vi "Message Handling Loop - Screenpop.vi"(8 "error in":errorcluster, 9 "Message Queues in":T1, 10 "User Event Bundle":T2) -> (0 "error out":errorcluster)   [LabVIEW 2018]
uses:
  Type Defs/User Events.ctl
  Support/Message Queue/All Message Queues.ctl
  Support/Message Queue/Message Cluster.ctl
  Type Defs/Screenpop Loop Data.ctl
  Type Defs/FGV States.ctl
  <vilib>/Utility/error.llb/Error Cluster From Error Code.vi
  <vilib>/ErrorRing/Error Ring.xnode
  Support/Message Queue/Message Queue.lvlib
  Support/User Events/User Events.lvlib
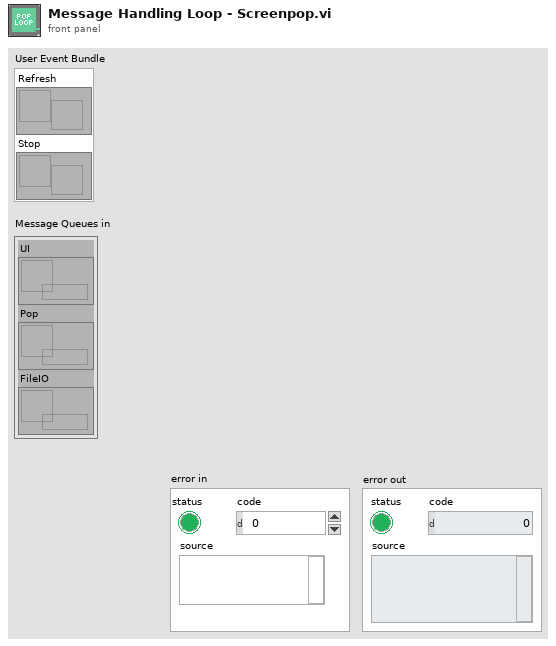
[diagram p1: front panel]
types:
  T1 = typedef "Message Queue.lvlib/All Message Queues.ctl" = cluster{"UI":refnum<queue>, "Pop":refnum<queue>, "FileIO":refnum<queue>}
  T2 = typedef "User Events.ctl" = cluster{"Refresh":refnum<user-event>, "Stop":refnum<user-event>}
  T3 = typedef "Screenpop Loop Data.ctl" = cluster{"Update List":i32[], "UI":refnum<queue>}
  T4 = typedef "FGV States.ctl" = enum16{"Initialize", "Merge", "Write", "Remove", "Read", "Clear"}
  T5 = typedef "SR Cluster.ctl" = cluster{"Color":u32, "SR Number":i32, "SR Status":T6, "Name":string, "Summary":string, "Last Updated":timestamp, "SR Type":string, "Service Level":string, "Days Open":dbl, "Creation Date":timestamp, "Owner":string, "Note":string}
  T6 = typedef "SR Status.ctl" = enum16{"Caller Abandoned", "Created in Error", "Expired", "Forum Resolved AE", "Forum Resolved Customer", "IN WORK", "IN WORK Collab with AES", "IN WORK Collab with PSE", "IN WORK Collab with SE", "IN WORK Customer Added Note", "IN WORK Escalation", "IN WORK Wait on Customer", "Open", "Potentially Resolved", "Presumed Resolved", "RMA Approved for Return", "RMA Closed", "RMA Closed - DOA", "RMA In Progress", "RMA Open", "RMA Waiting on Customer", "Resolved", "Passed Off"}
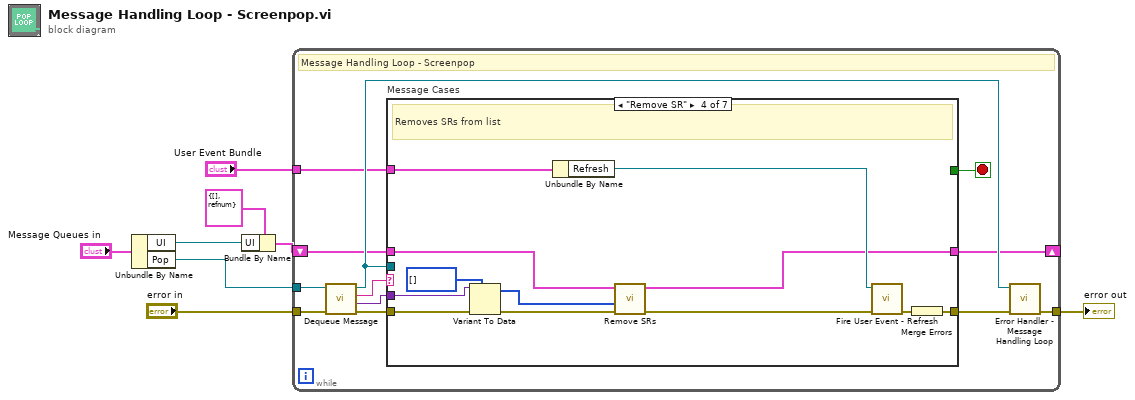
[diagram p0: block diagram]
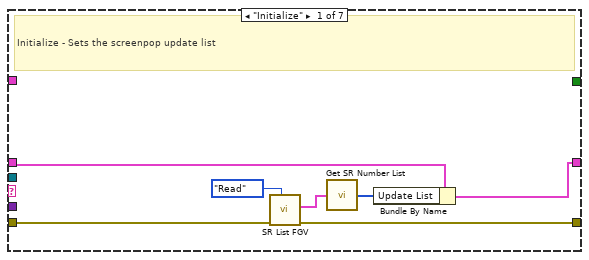
[diagram p2: hidden frame]
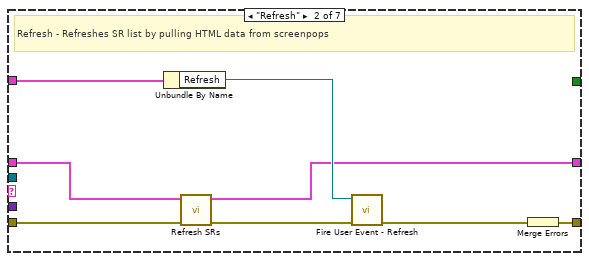
[diagram p3: hidden frame]
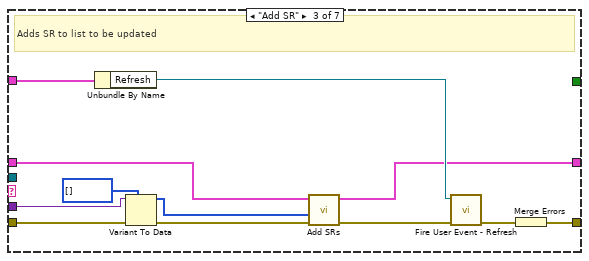
[diagram p4: hidden frame]
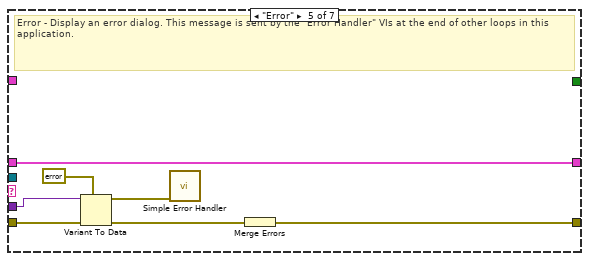
[diagram p5: hidden frame]
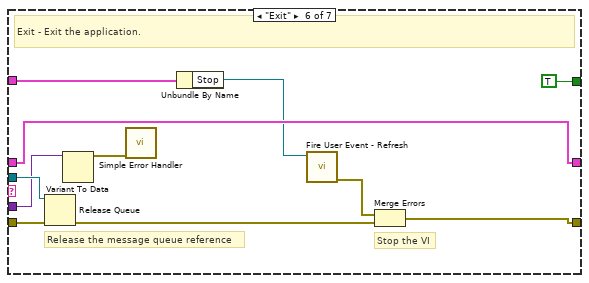
[diagram p6: hidden frame]
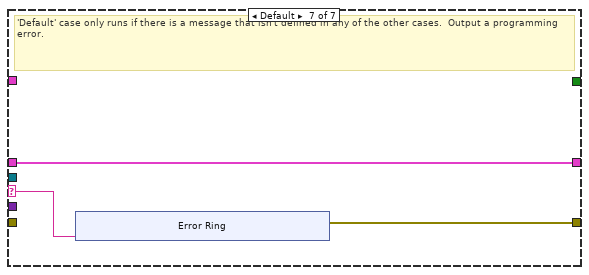
[diagram p7: hidden frame]
diagram:
  n1 = Unbundle By Name("Message Queues in") -> ("UI"=w5:refnum<queue>, "Pop"=w4:refnum<queue>)
  n2 = Bundle By Name(cluster=T3 {"Update List"=[], "UI"=refnum} ("Data Loop Data in"), "UI"=w5) -> (w7:T3)
  n3 = while {
    tunnel: w4 -> [w16]
    tunnel: [w14] -> w1
    shift-right: [w11] -> _
    shift-left: w7 -> [w12]
    tunnel: "error in" -> [w10]
    tunnel: "User Event Bundle" -> [w9]
    stop <- w20 stop-if-true
    # "Message Handling Loop - Screenpop"
    n4 = call "Dequeue Message.vi"("error in (no error)"=w10, "Message Queue"=w16) -> ("error out"=w19:errorcluster, "Message Data"=w17:variant, "Message"=w18:string, "dup Message Queue"=w15:refnum<queue>)  [unwired: 6 in]
    n5 = case "Message Cases" shown="\"Remove SR\"" w18 {
      selector: w18 -> [_ _ _ _ _ _ w79]
      tunnel: w15 -> [_ _ _ _ _ w77 _]
      tunnel: w19 -> [w21 w28 w44 w56 w66 w73 _]
      tunnel: [w23 w35 w47 w59 w61 w74 w80] -> w13
      tunnel: [_ _ _ _ _ TRUE _] -> w20
      tunnel: w17 -> [_ _ w46 w58 w65 w71 _]
      tunnel: w12 -> [w22 w29 w40 w51 w60 w70 w78]
      tunnel: [w27 w31 w39 w49 w60 w70 w78] -> w11
      tunnel: w9 -> [_ w34 w43 w55 _ w69 _]
      frame "Initialize" {
        # "Initialize - Sets the screenpop update list"
        n6 = call "SR List FGV.vi"("Operation"=FGV_States."Read", "Error In"=w21) -> ("Error Out"=w23:errorcluster, "list out"=w25:T5[])  [unwired: 8 in]
        n7 = call "Get SR Number List.vi"("list in"=w25) -> ("SR number array out"=w26:i32[])  [unwired: 4 in]
        n8 = Bundle By Name(cluster=w22, "Update List"=w26) -> (w27:T3)
      }
      frame "Refresh" {
        # "Refresh - Refreshes SR list by pulling HTML data from screenpops"
        n9 = Unbundle By Name(w34) -> ("Refresh"=w33:refnum<user-event>)
        n10 = call "Refresh SRs.vi"("error in"=w28, "Data Loop Data in"=w29) -> ("error out"=w30:errorcluster, "Data Loop Data out"=w31:T3)  [unwired: 8 in]
        n11 = call "Fire User Event - Refresh.vi"("error in (no error)"=w30, "Refresh"=w33) -> ("error out"=w32:errorcluster)  [unwired: 9 in]
        n12 = Merge Errors(w32) -> (w35:errorcluster)
      }
      frame "Add SR" {
        # "Adds SR to list to be updated"
        n13 = Unbundle By Name(w43) -> ("Refresh"=w42:refnum<user-event>)
        n14 = Variant To Data(error in=w44, type=i32[] [], Variant=w46) -> (data=w36:i32[], error out=w37:errorcluster)
        n15 = call "Add SRs.vi"("error in"=w37, "entered SRs in"=w36, "Data Loop Data in"=w40) -> ("error out"=w38:errorcluster, "Data Loop Data out"=w39:T3)  [unwired: 7 in]
        n16 = call "Fire User Event - Refresh.vi"("error in (no error)"=w38, "Refresh"=w42) -> ("error out"=w41:errorcluster)  [unwired: 9 in]
        n17 = Merge Errors(w41) -> (w47:errorcluster)
      }
      frame "Remove SR" {
        # "Removes SRs from list"
        n18 = Variant To Data(error in=w56, type=i32[] [], Variant=w58) -> (data=w52:i32[], error out=w50:errorcluster)
        n19 = Unbundle By Name(w55) -> ("Refresh"=w54:refnum<user-event>)
        n20 = call "Remove SRs.vi"("error in (no error)"=w50, "Array"=w52, "Data Loop Data in"=w51) -> ("error out"=w48:errorcluster, "Data Loop Data out"=w49:T3)  [unwired: 7 in]
        n21 = call "Fire User Event - Refresh.vi"("error in (no error)"=w48, "Refresh"=w54) -> ("error out"=w53:errorcluster)  [unwired: 9 in]
        n22 = Merge Errors(w53) -> (w59:errorcluster)
      }
      frame "Error" {
        # "Error - Display an error dialog. This message is sent by the \"Error Handler\" VIs at the end of other loops in this application."
        n23 = Variant To Data(error in=w66, type=errorcluster {"status"=FALSE, "code"=0, "source"=""} ("error constant"), Variant=w65) -> (data=w63:errorcluster, error out=w62:errorcluster)
        n24 = call <vilib>:"Simple Error Handler.vi"("error in (no error)"=w63) -> ()  [unwired: 4 in, 5 out]
        n25 = Merge Errors(w62) -> (w61:errorcluster)
      }
      frame "Exit" {
        # "Stop the VI"
        # "Release the message queue reference"
        # "Exit - Exit the application."
        n26 = Release Queue(queue=w77, error in (no error)=w73) -> (error out=w75:errorcluster)  [unwired: 1 in, 2 out]
        n27 = Variant To Data(Variant=w71) -> (data=w72:errorcluster)  [unwired: 2 in, 1 out]
        n28 = call <vilib>:"Simple Error Handler.vi"("error in (no error)"=w72) -> ()  [unwired: 4 in, 5 out]
        n29 = Unbundle By Name(w69) -> ("Stop"=w68:refnum<user-event>)
        n30 = call "Fire User Event - Refresh.vi"("Refresh"=w68) -> ("error out"=w67:errorcluster)  [unwired: 10 in]
        n31 = Merge Errors(w67, w75) -> (w74:errorcluster)
      }
      frame Default {
        # "'Default' case only runs if there is a message that isn't defined in any of the other cases.  Output a programming error."
        n32 = xnode "Error Ring"("parameter 0"=w79) -> ("error out"=w80:errorcluster)
      }
    }
    n33 = call "Error Handler - Message Handling Loop.vi"("error in (no error)"=w13, "Message Queue"=w15) -> ("dup error in"=w14:errorcluster)  [unwired: 8 in, 1 out]
  }
  "error out" <- w1
